vi "PPL_TRAJECTORY_EXECUTE_REL.vi"(8 "Init":bool, 9 "Max Wheel Speed M/S":dbl=2.5, 11 "Gyro Heading\nRAD":dbl) -> (0 "AtReference":bool, 1 "Position Error Ft":dbl, 2 "Right Speed Dmd M/S":dbl, 3 "Left Speed Dmd M/S":dbl)   [LabVIEW 2019]
uses:
  <vilib>/Rock Robotics/WPI/ThirdParty/JAS_Junk/TrajLib/Trajectory_Library.lvlib
  PPL_TRAJECTORY_GLOBALS.vi
  <vilib>/Rock Robotics/WPI/ThirdParty/MJansen/PathPlanner/PathPlanner24.lvlib
  <vilib>/Rock Robotics/WPI/ThirdParty/JAS_Junk/TrajLib/TypeDef/TRANSLATION2D.ctl
  <vilib>/Rock Robotics/WPI/ThirdParty/JAS_Junk/TrajLib/TypeDef/ROTATION2D.ctl
  <vilib>/Rock Robotics/WPI/ThirdParty/JAS_Junk/TrajLib/TypeDef/POSE2D.ctl
  <vilib>/Rock Robotics/WPI/ThirdParty/JAS_Junk/TrajLib/TypeDef/RAMSETE.ctl
  <vilib>/Rock Robotics/WPI/ThirdParty/MJansen/PathPlanner/TypeDef/PathPlannerTrajectory.ctl
  <vilib>/Rock Robotics/WPI/ThirdParty/MJansen/PathPlanner/TypeDef/PathPlannerTrajectoryState.ctl
  <vilib>/Rock Robotics/WPI/ThirdParty/MJansen/PathPlanner/TypeDef/PathPlannerPathConstraints.ctl
panel:
  out "PathPlannerTrajectory":T1 {"States"."TargetHolonomicRotation"."SIN" format="%13.4f"; "States"."TargetHolonomicRotation"."COS" format="%13.4f"; "States"."TargetHolonomicRotation"."VALUE" format="%13.4f"; "States"."Heading"."SIN" format="%13.4f"; "States"."Heading"."COS" format="%13.4f"; "States"."Heading"."VALUE" format="%13.4f"; "States"."PositionMeters"."Y" format="%14.3f"; "States"."PositionMeters"."X" format="%14.3f"}
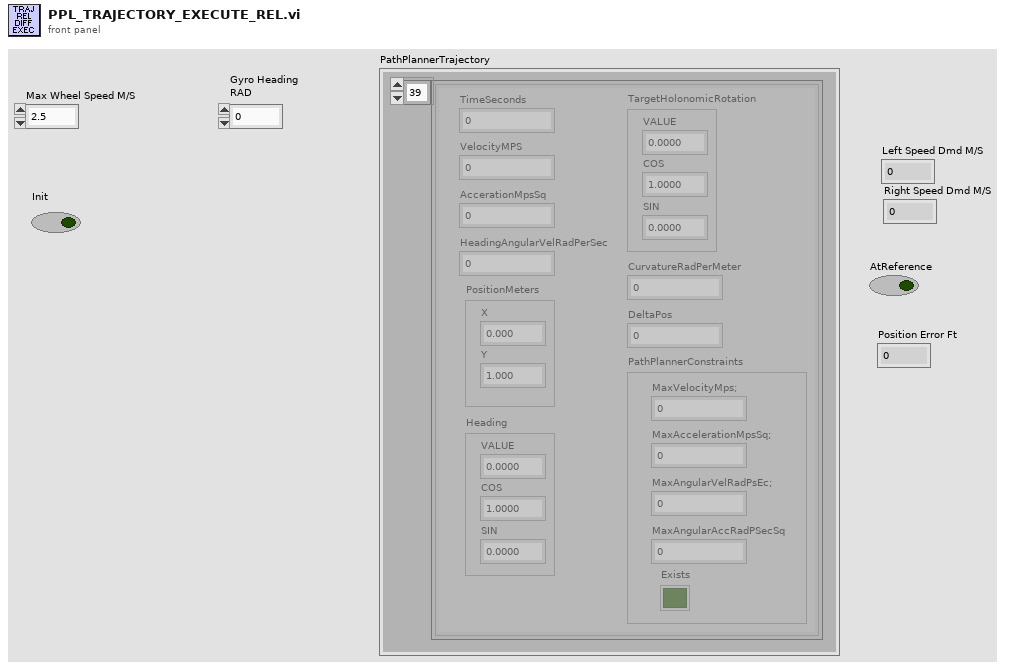
[diagram p1: front panel]
types:
  T1 = typedef "PathPlanner24.lvlib/PathPlannerTrajectory.ctl" = cluster{"States":T2[]}
  T2 = typedef "PathPlanner24.lvlib/PathPlannerTrajectoryState.ctl" = cluster{"TimeSeconds":dbl, "VelocityMPS":dbl, "AccerationMpsSq":dbl, "HeadingAngularVelRadPerSec":dbl, "PositionMeters":T3, "Heading":T4, "TargetHolonomicRotation":T4, "CurvatureRadPerMeter":dbl, "PathPlannerConstraints":T5, "DeltaPos":dbl}
  T3 = typedef "Trajectory_Library.lvlib/TRANSLATION2D.ctl" = cluster{"X":dbl, "Y":dbl}
  T4 = typedef "Trajectory_Library.lvlib/ROTATION2D.ctl" = cluster{"VALUE":dbl, "COS":dbl, "SIN":dbl}
  T5 = typedef "PathPlanner24.lvlib/PathPlannerPathConstraints.ctl" = cluster{"MaxVelocityMps;":dbl, "MaxAccelerationMpsSq;":dbl, "MaxAngularVelRadPsEc;":dbl, "MaxAngularAccRadPSecSq":dbl, "Exists":bool}
  T6 = typedef "Trajectory_Library.lvlib/POSE2D.ctl" = cluster{"TRANSLATION":T3, "ROTATION":T4}
  T7 = typedef "Trajectory_Library.lvlib/DIFF_DRIVE_KINEMATICS.ctl" = cluster{"TrackWidth_Meters":dbl}
  T8 = typedef "Trajectory_Library.lvlib/LTV_UNICYCLE_CONTROLLER_MODEL_PARAMS.CTL" = cluster{"Max linear ctrl effort M/S":dbl, "Max angular ctrl effort Rad/S":dbl, "Max Heading Meas Tol Rad":dbl, "Max X Pos Meas Tol M":dbl, "Max Y Pos Meas Tol M":dbl, "Max Linear Vel M/S":dbl}
  T9 = typedef "Trajectory_Library.lvlib/LTV_UNICYCLE_CONTROLLER_TOLERANCE.CTL" = cluster{"Max Heading Tolerance Rad":dbl, "Max X Tolerance M":dbl, "Max Y Tolerance M":dbl}
  T10 = typedef "Trajectory_Library.lvlib/RAMSETE.ctl" = cluster{"B":dbl, "Zeta":dbl, "poseTolerance":T6, "poseError":T6, "Enabled":bool}
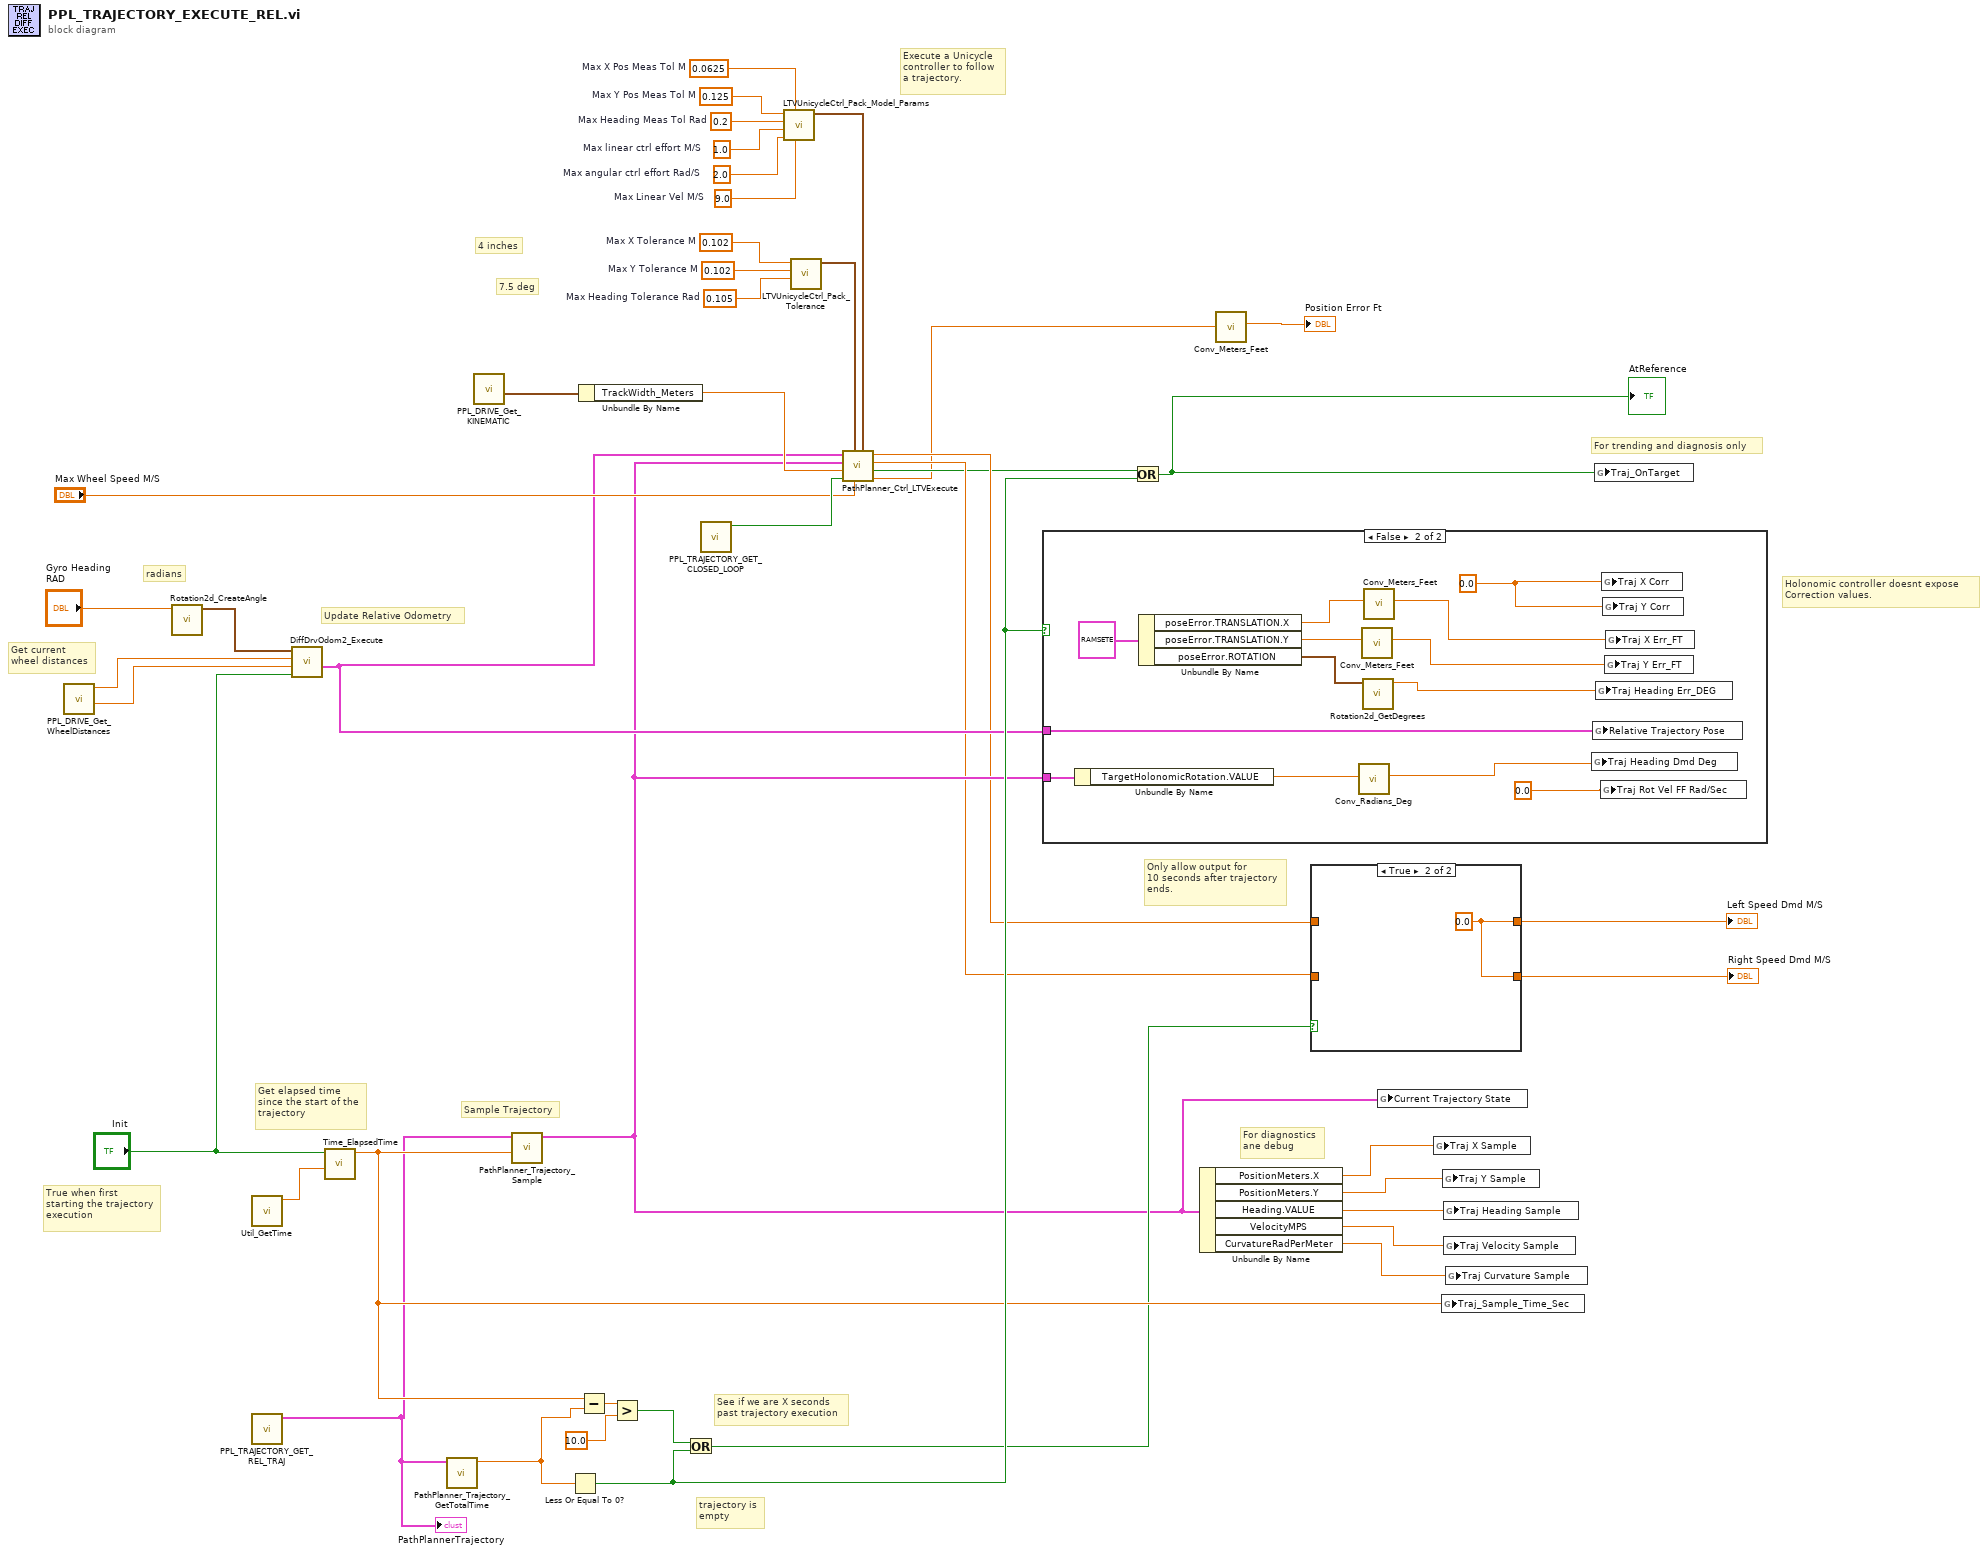
[diagram p0: block diagram]
diagram:
  w18 = 0.102  # Max X Tolerance M
  w17 = 0.102  # Max Y Tolerance M
  w16 = 0.105  # Max Heading Tolerance Rad
  w15 = 0.125  # Max Y Pos Meas Tol M
  w14 = 0.2  # Max Heading Meas Tol Rad
  w13 = 1.0  # Max linear ctrl effort M/S
  w12 = 2.0  # Max angular ctrl effort Rad/S
  w11 = 0.0625  # Max X Pos Meas Tol M
  w10 = 9.0  # Max Linear Vel M/S
  # "Execute a Unicycle\ncontroller to follow\na trajectory."
  # "4 inches"
  # "7.5 deg"
  # "Get current \nwheel distances"
  # "Update Relative Odometry"
  # "radians"
  # "trajectory is \nempty"
  # "True when first\nstarting the trajectory\nexecution"
  # "Get elapsed time\nsince the start of the\ntrajectory"
  # "Holonomic controller doesnt expose\nCorrection values."
  # "For trending and diagnosis only"
  # "For diagnostics\nane debug"
  # "Sample Trajectory"
  # "See if we are X seconds \npast trajectory execution"
  # "Only allow output for\n10 seconds after trajectory\nends."
  n1 = call "PPL_DRIVE_Get_WheelDistances.vi"() -> ("Right Wheel Dist M"=w26:dbl, "Left Wheel Dist M"=w27:dbl)  [unwired: 10 in]
  n2 = call <vilib>:"Rotation2d_CreateAngle.vi"("Angle"="Gyro Heading\nRAD") -> ("ROTATION"=w29:T4)  [unwired: 10 in]
  n3 = call <vilib>:"Util_GetTime.vi"() -> ("FPGA_Time_Seconds"=w42:dbl)  [unwired: 9 in, 2 out]
  n4 = call "PPL_TRAJECTORY_GET_REL_TRAJ.vi"() -> ("Relative_Trajectory"=w31:T1)  [unwired: 11 in]
  "PathPlannerTrajectory" <- w31
  n5 = call <vilib>:"DiffDrvOdom2_Execute.vi"("Init / Reset"="Init", "Right Distance M"=w26, "Left Distance M"=w27, "Gyro Reading"=w29) -> ("Pose Meters"=w6:T6)  [unwired: 6 in, 1 out]
  n6 = call <vilib>:"Time_ElapsedTime.vi"("PassthroughTime_SEC"=w42, "Reset"="Init") -> ("Elapsed Time Sec"=w33:dbl)  [unwired: 9 in]
  n7 = call <vilib>:"PathPlanner_Trajectory_GetTotalTime.vi"("PathPlannerTrajectory"=w31) -> ("TotalTimeSeconds"=w32:dbl)  [unwired: 10 in]
  n8 = call "PPL_DRIVE_Get_KINEMATIC.vi"() -> ("out DIFF_DRIVE_KINEMATICS"=w21:T7)  [unwired: 11 in]
  n9 = call <vilib>:"PathPlanner_Trajectory_Sample.vi"("Time"=w33, "PathPlannerTrajectory"=w31) -> ("PathPlannerState"=w5:T2)  [unwired: 9 in]
  n10 = Less Or Equal To 0?(x=w32) -> (x <= 0?=w34:bool)
  n11 = Unbundle By Name(w21) -> ("TrackWidth_Meters"=w9:dbl)
  n12 = Subtract(x=w33, y=w32) -> (x-y=w44:dbl)
  n13 = Greater?(x=w44, y=10.0) -> (0:w36:bool)
  n14 = Or(x=w36, y=w34) -> (x .or. y?=w23:bool)
  n15 = call "PPL_TRAJECTORY_GET_CLOSED_LOOP.vi"() -> ("AUTO_CLOSED_LOOP"=w8:bool)  [unwired: 11 in]
  n16 = call <vilib>:"LTVUnicycleCtrl_Pack_Model_Params.vi"("Max Linear Vel M/S"=w10, "Max X Pos Meas Tol M"=w11, "Max angular ctrl effort Rad/S"=w12, "Max linear ctrl effort M/S"=w13, "Max Heading Meas Tol Rad"=w14, "Max Y Pos Meas Tol M"=w15) -> ("LTV_Unicycle_Ctrl_Model _Params"=w20:T8)  [unwired: 5 in]
  n17 = call <vilib>:"LTVUnicycleCtrl_Pack_Tolerance.vi"("Max Heading Tolerance Rad"=w16, "Max Y Tolerance M"=w17, "Max X Tolerance M"=w18) -> ("LTV_Unicycle_Ctrl_Tolerance"=w19:T9)  [unwired: 8 in]
  n18 = call <vilib>:"PathPlanner_Ctrl_LTVExecute.vi"("LTV_Unicycle_Ctrl_Model"=w20, "Max Speed M/S"="Max Wheel Speed M/S", "LTV_Unicycle_Ctrl_Tolerance"=w19, "Enabled"=w8, "Track Width Meters"=w9, "PathPlannerState"=w5, "Current Pose SI"=w6) -> ("Position Error M"=w1:dbl, "At Reference"=w2:bool, "Normalized Right Wheel Dmd M/S"=w3:dbl, "Normalized Left Wheel Dmd M/S"=w4:dbl)  [unwired: 1 in]
  n19 = case shown="False" w34 {
    tunnel: w6 -> [_ w48]
    tunnel: w5 -> [_ w51]
    frame True {
    }
    frame False {
      w57 = 0.0 ("Y Corr")
      n20 = Unbundle By Name(w51) -> ("TargetHolonomicRotation.VALUE"=w50:dbl)
      n21 = Unbundle By Name(T10 {"B"=2.0, "Zeta"=0.7, "poseTolerance"={"TRANSLATION"={"X"=0.0, "Y"=0.0}, "ROTATION"={"VALUE"=0.0, "COS"=1.0, "SIN"=0.0}}, "poseError"={"TRANSLATION"={"X"=0.0, "Y"=0.0}, "ROTATION"={"VALUE"=0.0, "COS"=1.0, "SIN"=0.0}}, "Enabled"=TRUE} ("outRAMSETE")) -> ("poseError.TRANSLATION.X"=w53:dbl, "poseError.TRANSLATION.Y"=w52:dbl, "poseError.ROTATION"=w46:T4)
      n22 = call <vilib>:"Conv_Radians_Deg.vi"("Radians"=w50) -> ("Degrees"=w49:dbl)  [unwired: 10 in]
      n23 = call <vilib>:"Conv_Meters_Feet.vi"("Meters"=w52) -> ("Feet"=w56:dbl)  [unwired: 10 in]
      n24 = call <vilib>:"Rotation2d_GetDegrees.vi"("in ROTATION"=w46) -> ("AngleDegrees"=w47:dbl)  [unwired: 10 in]
      n25 = call <vilib>:"Conv_Meters_Feet.vi"("Meters"=w53) -> ("Feet"=w55:dbl)  [unwired: 10 in]
      n26 = global write "PPL_TRAJECTORY_GLOBALS.vi" "Traj Heading Dmd Deg"(w49) -> ()
      n27 = global write "PPL_TRAJECTORY_GLOBALS.vi" "Relative Trajectory Pose"(w48) -> ()
      n28 = global write "PPL_TRAJECTORY_GLOBALS.vi" "Traj Heading Err_DEG"(w47) -> ()
      n29 = global write "PPL_TRAJECTORY_GLOBALS.vi" "Traj Rot Vel FF Rad/Sec"(0.0 ("Traj Heading Dmd Deg")) -> ()
      n30 = global write "PPL_TRAJECTORY_GLOBALS.vi" "Traj X Corr"(w57) -> ()
      n31 = global write "PPL_TRAJECTORY_GLOBALS.vi" "Traj Y Corr"(w57) -> ()
      n32 = global write "PPL_TRAJECTORY_GLOBALS.vi" "Traj Y Err_FT"(w56) -> ()
      n33 = global write "PPL_TRAJECTORY_GLOBALS.vi" "Traj X Err_FT"(w55) -> ()
    }
  }
  n34 = Or(x=w2, y=w34) -> (x .or. y?=w35:bool)
  "AtReference" <- w35
  n35 = Unbundle By Name(w5) -> ("PositionMeters.X"=w41:dbl, "PositionMeters.Y"=w40:dbl, "Heading.VALUE"=w39:dbl, "VelocityMPS"=w38:dbl, "CurvatureRadPerMeter"=w37:dbl)
  n36 = call <vilib>:"Conv_Meters_Feet.vi"("Meters"=w1) -> ("Feet"=→"Position Error Ft":dbl)  [unwired: 10 in]
  n37 = case shown="True" w23 {
    tunnel: w4 -> [w59 _]
    tunnel: [w59 w60] -> w25
    tunnel: w3 -> [w58 _]
    tunnel: [w58 w60] -> w24
    frame False {
    }
    frame True {
      w60 = 0.0 ("vX")
    }
  }
  "Left Speed Dmd M/S" <- w25
  "Right Speed Dmd M/S" <- w24
  n38 = global write "PPL_TRAJECTORY_GLOBALS.vi" "Current Trajectory State"(w5) -> ()
  n39 = global write "PPL_TRAJECTORY_GLOBALS.vi" "Traj X Sample"(w41) -> ()
  n40 = global write "PPL_TRAJECTORY_GLOBALS.vi" "Traj_Sample_Time_Sec"(w33) -> ()
  n41 = global write "PPL_TRAJECTORY_GLOBALS.vi" "Traj Y Sample"(w40) -> ()
  n42 = global write "PPL_TRAJECTORY_GLOBALS.vi" "Traj Heading Sample"(w39) -> ()
  n43 = global write "PPL_TRAJECTORY_GLOBALS.vi" "Traj Velocity Sample"(w38) -> ()
  n44 = global write "PPL_TRAJECTORY_GLOBALS.vi" "Traj Curvature Sample"(w37) -> ()
  n45 = global write "PPL_TRAJECTORY_GLOBALS.vi" "Traj_OnTarget"(w35) -> ()
